vi "Configuration Process.vi"(8 "error in (no error)":errorcluster, 11 "View Model":T1) -> (0 "error out":errorcluster)   [LabVIEW 2017]
doc: "Contains operations of Configuration DB process of Car Wash Controller"
uses:
  View Model/Controls/View Model.ctl
  View Model/Controls/Shared Model.ctl
  Error Handler/Controls/Error Model.ctl
  Error Handler/Controls/Error Data.ctl
  Error Handler/Controls/Error Level.ctl
  Controls/Config Model.ctl
  Controls/Config Record.ctl
  Controls/Config Data.ctl
  Controls/Config Command.ctl
  Controller/Controls/Controler Model.ctl
  Views/Entry Console View/Controls/Entry Console - Wash Steps.ctl
  Controller/Controls/Controller - Overhead.ctl
  Controller/Controls/Controller - States.ctl
  Controller/Controls/Controller - Wash Step.ctl
  Views/Vehicle Position View/Controls/Vehicle - Station Enum.ctl
  Controller/Controls/Controller - Event.ctl
  Controller/Controls/Controller - Commands.ctl
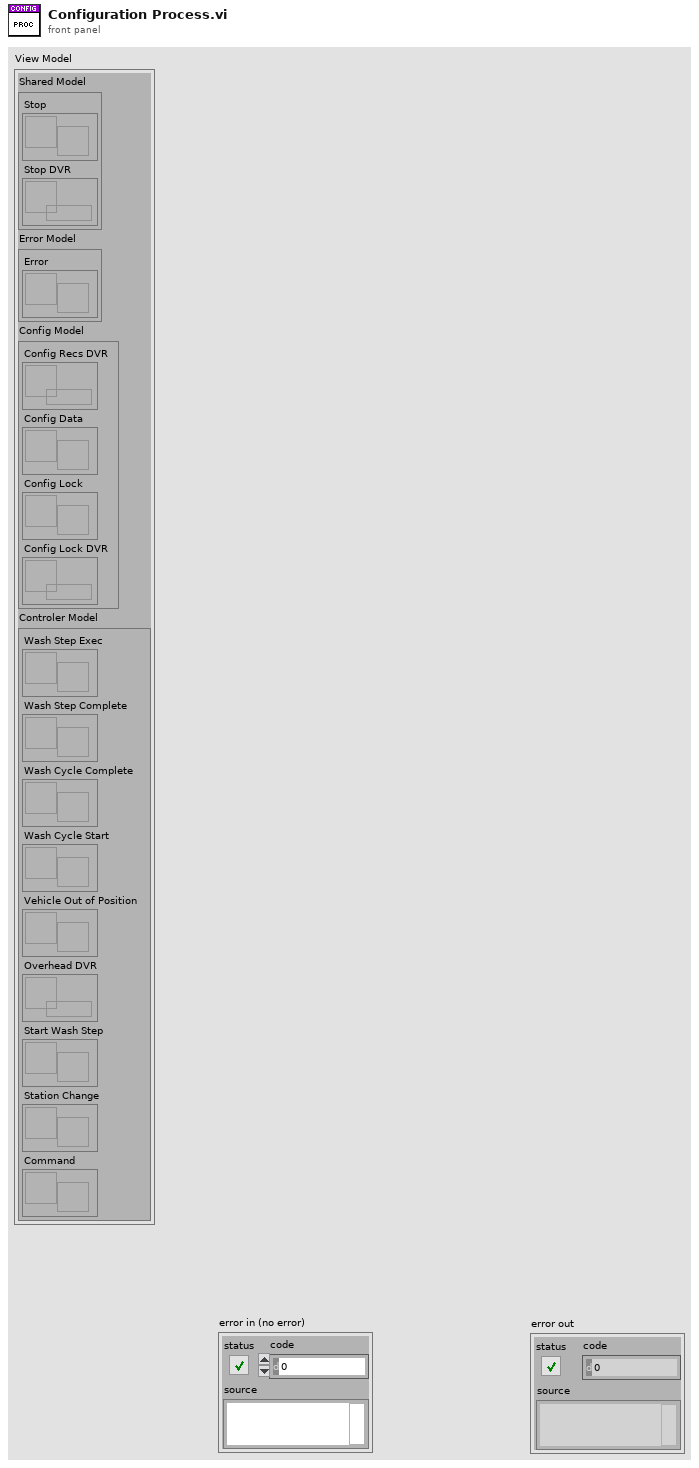
[diagram p1: front panel]
types:
  T1 = typedef "View Model.ctl" = cluster{"Shared Model":T2, "Error Model":T3, "Config Model":T4, "Controler Model":T5}
  T2 = typedef "Shared Model.ctl" = cluster{"Stop":refnum<user-event>, "Stop DVR":refnum<data-value>}
  T3 = typedef "Error Model.ctl" = cluster{"Error":refnum<user-event>}
  T4 = typedef "Config Model.ctl" = cluster{"Config Recs DVR":refnum<data-value>, "Config Data":refnum<user-event>, "Config Lock":refnum<user-event>, "Config Lock DVR":refnum<data-value>}
  T5 = typedef "Controler Model.ctl" = cluster{"Wash Step Exec":refnum<user-event>, "Wash Step Complete":refnum<user-event>, "Wash Cycle Complete":refnum<user-event>, "Wash Cycle Start":refnum<user-event>, "Vehicle Out of Position":refnum<user-event>, "Overhead DVR":refnum<data-value>, "Start Wash Step":refnum<user-event>, "Station Change":refnum<user-event>, "Command":refnum<user-event>}
  T6 = typedef "Config Record.ctl" = cluster{"Wash Step":string, "Station":string, "Step Duration":u32}
  T7 = typedef "Config Command.ctl" = enum16{"Read", "Query", "Insert", "Update"}
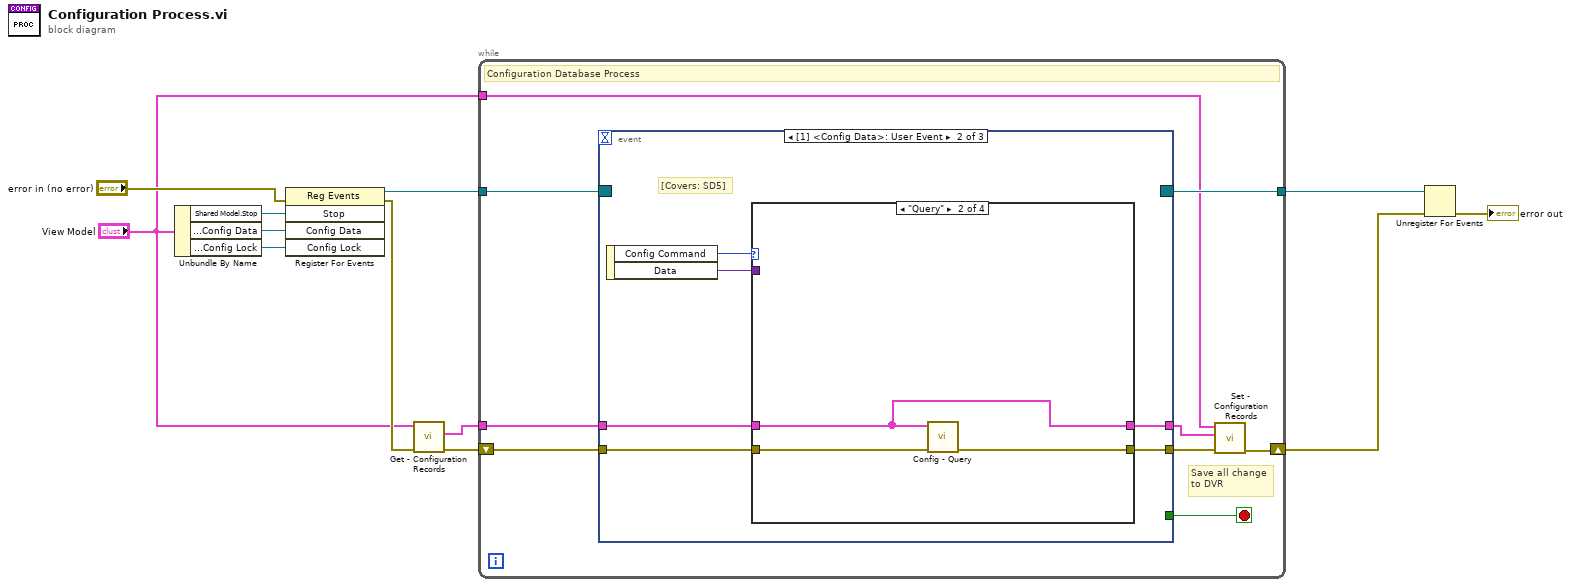
[diagram p0: block diagram]
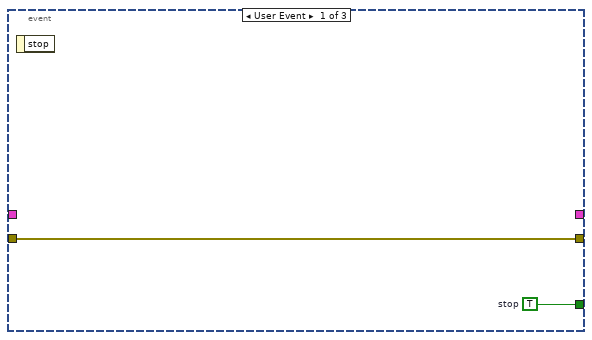
[diagram p2: hidden frame]
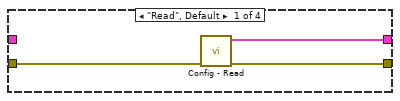
[diagram p3: hidden frame]
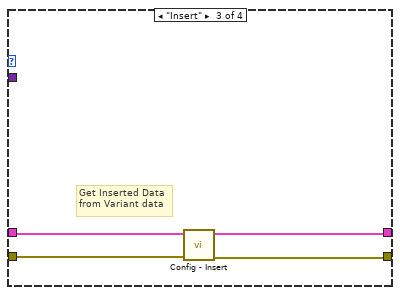
[diagram p4: hidden frame]
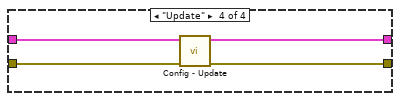
[diagram p5: hidden frame]
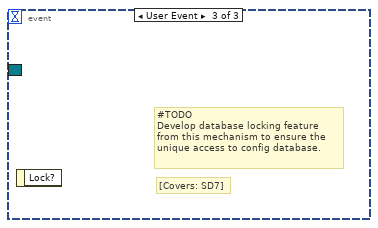
[diagram p6: hidden frame]
diagram:
  n1 = Unbundle By Name("View Model") -> ("Shared Model.Stop"=w12:refnum<user-event>, "Config Model.Config Data"=w6:refnum<user-event>, "Config Model.Config Lock"=w7:refnum<user-event>)
  n2 = register-events(error in="error in (no error)", w12, w6, w7) -> (reference out=w10:refnum<event-registration>, error out=w5:errorcluster)  [unwired: 1 in]
  n3 = call "Get - Configuration Records.vi"("error in (no error)"=w5, "View Model"="View Model") -> ("error out"=w4:errorcluster, "Config Records"=w3:T6[])  [unwired: 7 in, 1 out]
  n4 = while {
    tunnel: w10 -> [w21]
    shift-right: [w15] -> w2
    shift-left: w4 -> [w20]
    tunnel: [w18] -> w9
    tunnel: w3 -> [w17]
    tunnel: "View Model" -> [w13]
    stop <- w19 stop-if-true
    # "Save all change\nto DVR"
    # "Configuration Database Process"
    n5 = event shown="[1] <Config Data>: User Event" {
      selector: w21 -> [_ _ _]
      dyn-events: [_ _ _] -> w18
      timeout: _ -> [_ _ _]
      tunnel: w20 -> [w23 w25 _]
      tunnel: [w23 w24 _] -> w16
      tunnel: [w22 _ _] -> w19
      tunnel: w17 -> [_ w27 _]
      tunnel: [_ w26 _] -> w14
      event User Event {
        w22 = TRUE  # stop
        n6 = event-data() -> ()  [unwired: 1 in, 1 out]
      }
      event User Event {
        # "[Covers: SD5]"
        n7 = event-data() -> ("Config Command"=w29:T7, "Data"=w28:variant)  [unwired: 1 in]
        n8 = case shown="\"Query\"" w29 {
          tunnel: w28 -> [_ _ _ _]
          tunnel: w27 -> [_ w33 w36 w42]
          tunnel: [w32 w33 w37 w41] -> w26
          tunnel: w25 -> [w31 w35 w39 w43]
          tunnel: [w30 w34 w38 w40] -> w24
          frame "Read", Default {
            n9 = call "Config - Read.vi"("error in (no error)"=w31) -> ("error out"=w30:errorcluster, "Config Records"=w32:T6[])  [unwired: 9 in]
          }
          frame "Query" {
            n10 = call "Config - Query.vi"("error in (no error)"=w35, "Config Records"=w33) -> ("error out"=w34:errorcluster)  [unwired: 8 in, 1 out]
          }
          frame "Insert" {
            # "Get Inserted Data\nfrom Variant data"
            n11 = call "Config - Insert.vi"("error in (no error)"=w39, "Config Records"=w36) -> ("error out"=w38:errorcluster, "Config Records"=w37:T6[])  [unwired: 8 in]
          }
          frame "Update" {
            n12 = call "Config - Update.vi"("error in (no error)"=w43, "Config Records"=w42) -> ("error out"=w40:errorcluster, "Config Records"=w41:T6[])  [unwired: 8 in]
          }
        }
      }
      event User Event {
        # "[Covers: SD7]"
        # "#TODO\nDevelop database locking feature\nfrom this mechanism to ensure the\nunique access to config database."
        n13 = event-data() -> ()  [unwired: 1 in, 1 out]
      }
    }
    n14 = call "Set - Configuration Records.vi"("error in (no error)"=w16, "Config Records"=w14, "View Model"=w13) -> ("error out"=w15:errorcluster)  [unwired: 7 in, 1 out]
  }
  n15 = Unregister For Events(event registration refnum=w9, error in=w2) -> (error out=→"error out":errorcluster)
